vi "Init.vi"(8 "error in (no error)":errorcluster, 10 "index":i32, 11 "IC_1D_VIRef":refnum<class "NI_IC_1D_VIRef.lvclass">) -> (0 "error out":errorcluster, 3 "initialized IC_1D_VIRef":refnum<class "NI_IC_1D_VIRef.lvclass">)   [LabVIEW 2020, in "NI_PDE.lvlib" / "NI_IC_1D_VIRef.lvclass"]
uses:
  <vilib>/gmath/pde.llb/ICClass/IC_1D_VIRef/NI_IC_1D_VIRef.lvclass
  <vilib>/gmath/pde.llb/ICClass/Class Type.ctl
  <vilib>/gmath/pde.llb/ICClass/IC_1D_VIRef/NI_IC_1D_VIRef.lvclass/NI_IC_1D_VIRef.ctl
  <vilib>/gmath/pde.llb/ICClass/NI_IC.lvclass
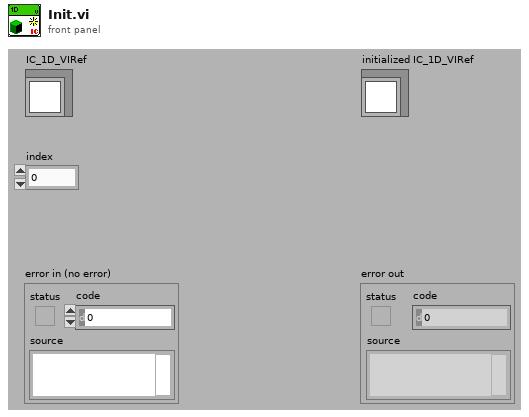
[diagram p1: front panel]
types:
  T1 = typedef "NI_PDE.lvlib/NI_IC.lvclass/Class Type.ctl" = i32
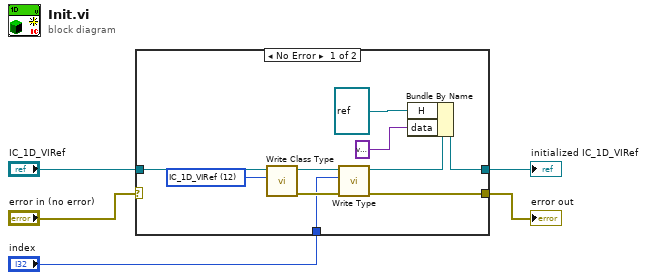
[diagram p0: block diagram]
diagram:
  n1 = case shown="No Error" "error in (no error)" {
    selector: "error in (no error)" -> [_ w17]
    tunnel: [w9 w16] -> w5
    tunnel: [w6 w17] -> w4
    tunnel: "IC_1D_VIRef" -> [w12 w16]
    tunnel: "index" -> [w11 _]
    frame No Error {
      w13 = T1 12 items=["IC"=0, "IC_1D"=10, "IC_1D_Numeric"=11, "IC_1D_VIRef"=12, "IC_2D"=20, "IC_2D_Numeric"=21, "IC_2D_VIRef"=22] ("IC class type")
      n2 = call-dynamic "Write Class Type.vi"("IC class type"=w13, "IC.lvclass in"=w12) -> ("error out"=w14:errorcluster, "IC.lvclass out"=w15:refnum<class "NI_IC_1D_VIRef.lvclass">)  [unwired: 1 in, 7 out]
      n3 = call-dynamic "Write Type.vi"("error in (no error)"=w14, "IC type"=w11, "IC.lvclass in"=w15) -> ("error out"=w6:errorcluster, "IC.lvclass out"=w10:refnum<class "NI_IC_1D_VIRef.lvclass">)  [unwired: 7 out]
      n4 = Bundle By Name(cluster=w10, "H"=refnum<vi> refnum ("G"), "data"=variant) -> (w9:refnum<class "NI_IC_1D_VIRef.lvclass">)
    }
    frame Error {
    }
  }
  "initialized IC_1D_VIRef" <- w5
  "error out" <- w4
